vi "Track peg with Pixy.vi"() -> (1 "sees peg":bool, 2 "y output":dbl, 3 "x output":dbl)   [LabVIEW 2016]
uses:
  Robot Global Data.vi
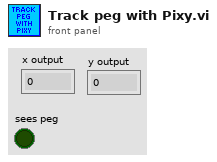
[diagram p1: front panel]
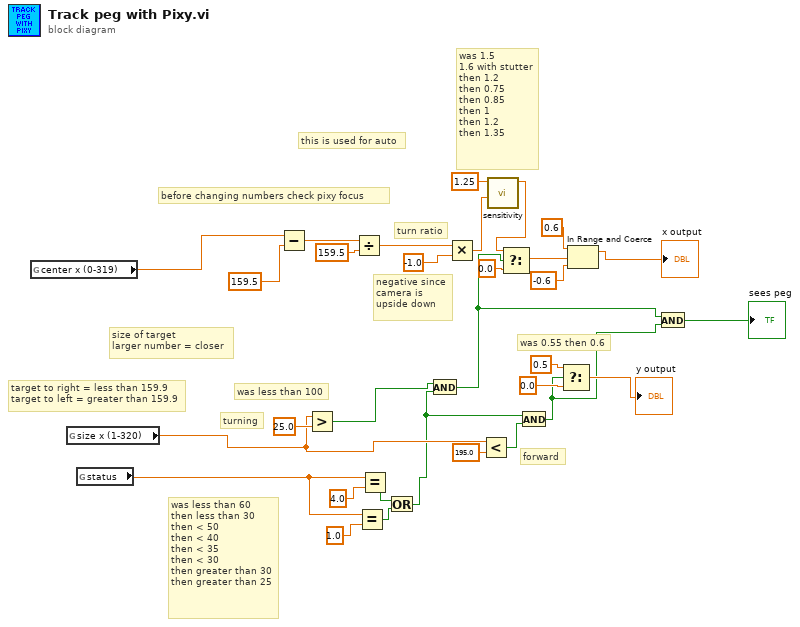
[diagram p0: block diagram]
diagram:
  # "was 1.5\n1.6 with stutter\nthen 1.2\nthen 0.75\nthen 0.85\nthen 1\nthen 1.2\nthen 1.35"
  # "was 0.55 then 0.6"
  # "this is used for auto"
  # "negative since\ncamera is \nupside down"
  # "was less than 100"
  # "before changing numbers check pixy focus"
  # "forward"
  # "turning"
  # "size of target\nlarger number = closer"
  # "turn ratio"
  # "was less than 60\nthen less than 30\nthen < 50\nthen < 40\nthen < 35\nthen < 30\nthen greater than 30\nthen greater than 25"
  # "target to right = less than 159.9\ntarget to left = greater than 159.9"
  n1 = global read "Robot Global Data.vi" "center x (0-319)"() -> (w18:dbl)
  n2 = global read "Robot Global Data.vi" "size x (1-320)"() -> (w19:dbl)
  n3 = global read "Robot Global Data.vi" "status"() -> (w11:dbl)
  n4 = Subtract(x=w18, y=159.5) -> (x-y=w27:dbl)
  n5 = Greater?(x=w19, y=25.0) -> (0:w23:bool)
  n6 = Divide(x=w27, y=159.5) -> (x/y=w24:dbl)
  n7 = Equal?(x=w11, y=1.0) -> (x = y?=w9:bool)
  n8 = Equal?(x=w11, y=4.0) -> (x = y?=w10:bool)
  n9 = Or(x=w10, y=w9) -> (x .or. y?=w8:bool)
  n10 = And(x=w23, y=w8) -> (x .and. y?=w16:bool)
  n11 = Multiply(x=w24, y=-1.0) -> (x*y=w7:dbl)
  n12 = Less?(x=w19, y=195.0) -> (x < y?=w20:bool)
  n13 = call "sensitivity.vi"("x"=w7, "sensitivity"=1.25) -> ("scaled value"=w6:dbl)  [unwired: 9 in]
  n14 = Select(t=w6, s=w16, f=0.0) -> (s? t:f=w4:dbl)
  n15 = And(x=w8, y=w20) -> (x .and. y?=w15:bool)
  n16 = Select(t=0.5, s=w15, f=0.0) -> (s? t:f=→"y output":dbl)
  n17 = In Range and Coerce(upper limit=0.6, x=w4, lower limit=-0.6 ("x")) -> (coerced(x)=→"x output":dbl)  [unwired: 1 out]
  n18 = And(x=w16, y=w15) -> (x .and. y?=→"sees peg":bool)
